vi "Write Update Rate (4Hz-100Hz).vi"(8 "error in (no error)":errorcluster, 10 "Update Rate (4Hz-100Hz)":u8=4 min=4 max=100 step=1, 11 "navX - Base in":refnum<class "navX - Interface.lvclass">) -> (0 "error out":errorcluster, 3 "navX - Base out":refnum<class "navX - Interface.lvclass">)   [LabVIEW 2015, in "navX Library v3.lvlib" / "navX - Interface.lvclass"]
uses:
  navX - Interface.lvclass
  navX - Interface.lvclass/navX - Interface.ctl
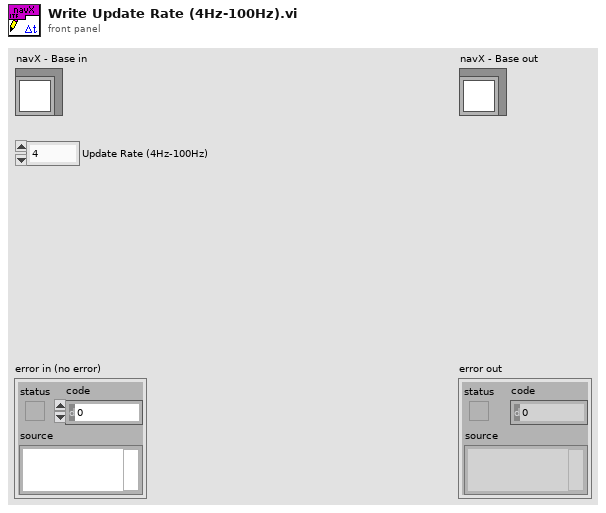
[diagram p1: front panel]
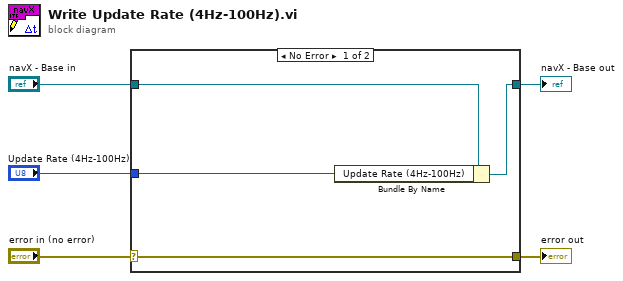
[diagram p0: block diagram]
diagram:
  n1 = case shown="No Error" "error in (no error)" {
    selector: "error in (no error)" -> [w9 w10]
    tunnel: [w9 w10] -> w4
    tunnel: [w7 w11] -> w2
    tunnel: "navX - Base in" -> [w8 w11]
    tunnel: "Update Rate (4Hz-100Hz)" -> [w6 _]
    frame No Error {
      n2 = Bundle By Name(cluster=w8, "Update Rate (4Hz-100Hz)"=w6) -> (w7:refnum<class "navX - Interface.lvclass">)
    }
    frame Error {
    }
  }
  "error out" <- w4
  "navX - Base out" <- w2
